vi "HostFormatXYGraphs (1).vi"(11 "CurrentState":T1) -> (1 "Acceleration Graph":cluster{dbl[], dbl[]}, 2 "Speed Graph":cluster{dbl[], dbl[]}, 3 "Distance Graph":cluster{dbl[], dbl[]})   [LabVIEW 2017]
uses:
  RTControl/StateList.ctl
  Sensors/DataStreamIndex.ctl
  HostDataGLOBAL.vi
  HostCurrentTimeGLOBAL.vi
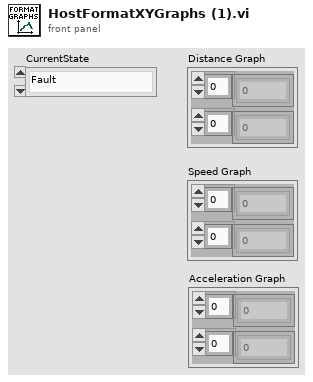
[diagram p1: front panel]
types:
  T1 = typedef "StateList.ctl" = enum16{"Fault", "Idle", "Ready", "Pushing", "Coast", "Braking"}
  T2 = typedef "DataStreamIndex.ctl" = enum16{"SuspensionPT (PSI)", "MagBrakePT (PSI)", "Baby HPPT (PSI)", "BigRight HPPT (PSI)", "BigLeft HPPT (PSI)", "HallEffect FrontLeft (V)", "HallEffect FrontRight (V)", "HallEffect BackRight (V)", "HallEffect BackLeft (V)", "LinearPot FrontRight (V)", "LinearPot FrontLeft (V)", "LinearPot BackRight (V)", "LinearPot BackLeft (V)", "Speed (m/s)", "Distance (m)", "Piezo (V)", "Battery Voltage (V)", "Battery Current", "Battery Temperature (C)", "cRIO Temperature (C)", "Right Big Tank Temperature (C)", "Left Big Tank Temperature (C)", "Baby Tank Temperature (C)", "Right Manifold Temperature (C)", "Left Manifold Temperature (C)", "IMU Acceleration (m/s2)", "IMU Pressure (Pa)", "IMU Temperature (C)"}
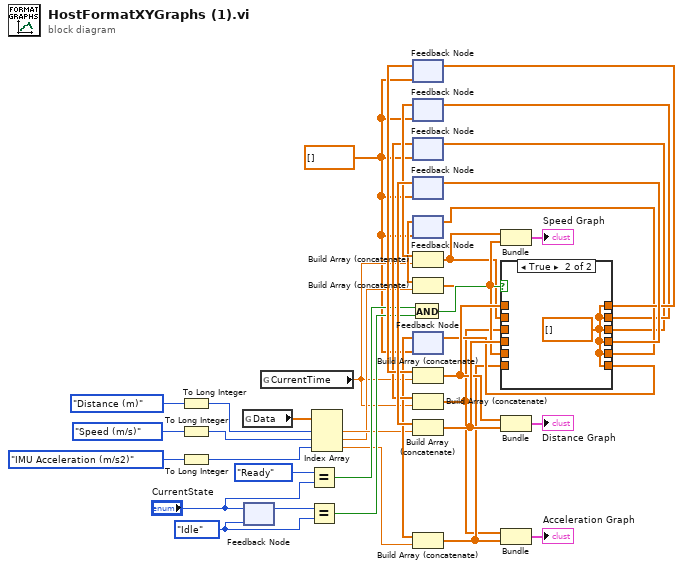
[diagram p0: block diagram]
diagram:
  w25 = StateList."Idle" ("CurrentState")
  w3 = dbl[] []
  n1 = To Long Integer(number=DataStreamIndex."Distance (m)" ("Data Stream Index")) -> (32bit integer=w39:i32)
  n2 = To Long Integer(number=DataStreamIndex."Speed (m/s)" ("Data Stream Index")) -> (32bit integer=w40:i32)
  n3 = To Long Integer(number=DataStreamIndex."IMU Acceleration (m/s2)" ("Data Stream Index")) -> (32bit integer=w2:i32)
  n4 = global read "HostDataGLOBAL.vi" "Data"() -> (w38:dbl[])
  n5 = feedback #1(w25) -> (w26:T1)
  n6 = feedback-in #1("CurrentState") -> ()
  n7 = global read "HostCurrentTimeGLOBAL.vi" "CurrentTime"() -> (w4:dbl)
  n8 = Equal?(x=StateList."Ready", y="CurrentState") -> (x = y?=w22:bool)
  n9 = Equal?(x=w26, y=w25) -> (x = y?=w21:bool)
  n10 = Index Array(array=w38, index #1=w39, index #2=w40, index #3=w2) -> (element #1=w7:dbl, element #2=w6:dbl, element #3=w5:dbl)
  n11 = And(x=w22, y=w21) -> (x .and. y?=w20:bool)
  n12 = feedback #2(w3) -> (w33:dbl[])
  n13 = feedback #3(w3) -> (w32:dbl[])
  n14 = feedback #4(w3) -> (w30:dbl[])
  n15 = feedback #5(w3) -> (w34:dbl[])
  n16 = feedback #6(w3) -> (w31:dbl[])
  n17 = Build Array (concatenate)(w32, w4) -> (w13:dbl[])
  n18 = Build Array (concatenate)(w31, w6) -> (w15:dbl[])
  n19 = feedback #7(w3) -> (w29:dbl[])
  n20 = Build Array (concatenate)(w33, w4) -> (w17:dbl[])
  n21 = Build Array (concatenate)(w30, w4) -> (w9:dbl[])
  n22 = Build Array (concatenate)(w34, w7) -> (w19:dbl[])
  n23 = Build Array (concatenate)(w29, w5) -> (w10:dbl[])
  n24 = Bundle(w13, w15) -> (→"Speed Graph":cluster{dbl[], dbl[]})  [unwired: 1 in]
  n25 = case shown="True" w20 {
    tunnel: w19 -> [w46 _]
    tunnel: [w46 w47] -> w18
    tunnel: w17 -> [w45 _]
    tunnel: [w45 w47] -> w16
    tunnel: w15 -> [w44 _]
    tunnel: [w44 w47] -> w14
    tunnel: w13 -> [w43 _]
    tunnel: [w43 w47] -> w12
    tunnel: [w42 w47] -> w11
    tunnel: w10 -> [w42 _]
    tunnel: w9 -> [w41 _]
    tunnel: [w41 w47] -> w8
    frame False {
    }
    frame True {
      w47 = dbl[] []
    }
  }
  n26 = feedback-in #2(w16) -> ()
  n27 = feedback-in #3(w12) -> ()
  n28 = feedback-in #4(w8) -> ()
  n29 = feedback-in #5(w18) -> ()
  n30 = feedback-in #6(w14) -> ()
  n31 = feedback-in #7(w11) -> ()
  n32 = Bundle(w17, w19) -> (→"Distance Graph":cluster{dbl[], dbl[]})  [unwired: 1 in]
  n33 = Bundle(w9, w10) -> (→"Acceleration Graph":cluster{dbl[], dbl[]})  [unwired: 1 in]
